vi "test Future Already Completed if Resolved after Timeout.vi"(8 "error in (no error)":errorcluster, 11 "TestCase in":refnum<class "Result Tests.lvclass">) -> (0 "error out":errorcluster, 3 "TestCase out":refnum<class "Result Tests.lvclass">)   [LabVIEW 2017, in "Result Tests.lvclass"]
uses:
  Result Tests.lvclass
  <vilib>/addons/_JKI Toolkits/VI Tester/TestCase.llb/TestCase.lvclass
  Futures/Result/Result.lvclass
  C:/Program Files (x86)/National Instruments/LabVIEW 2017/vi.lib/addons/_JKI Toolkits/VI Tester/TestCase.llb/TestCase.lvclass
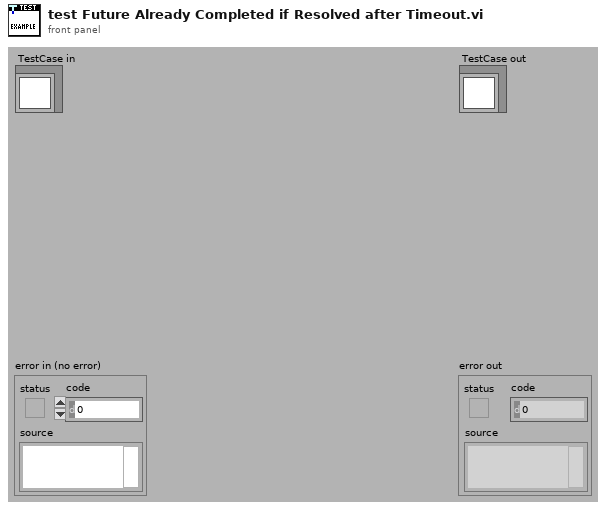
[diagram p1: front panel]
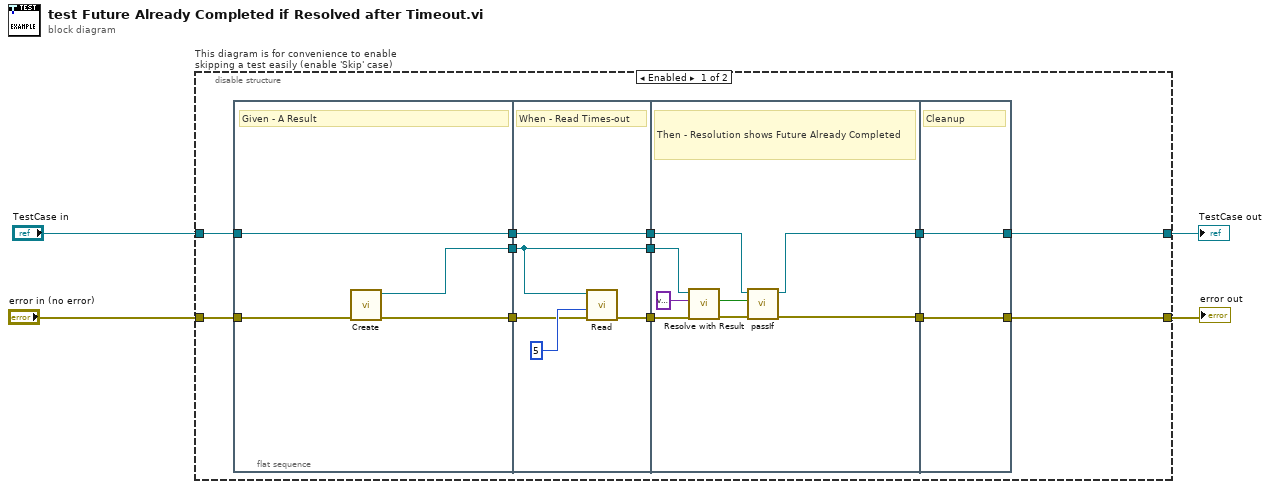
[diagram p0: block diagram]
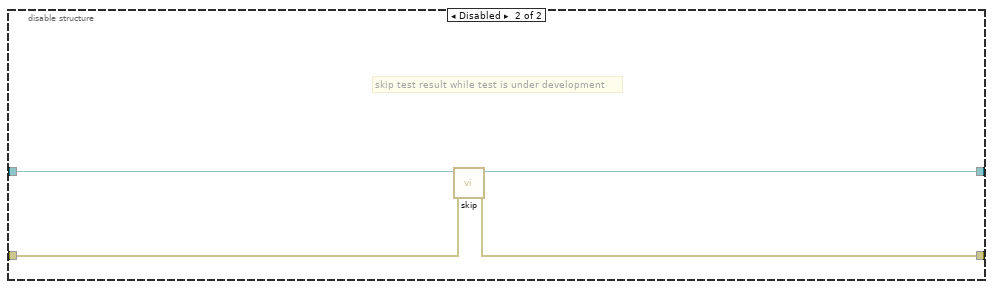
[diagram p2: hidden frame]
diagram:
  n1 = disable-structure "This diagram is for convenience to enable skipping a test easily (enable 'Skip' case)" shown="Enabled" {
    disable-tunnel: "TestCase in" -> [w11 w39]
    disable-tunnel: [w9 w37] -> w1
    disable-tunnel: [w8 w38] -> w3
    disable-tunnel: "error in (no error)" -> [w10 w36]
    frame Enabled {
      n2 = flat-sequence {
        tunnel: w10 -> [w19]
        tunnel: w11 -> [w20]
        tunnel: [w20] -> w16
        tunnel: [w18] -> w15
        tunnel: [w17] -> w7
        tunnel: [w25] -> w14
        tunnel: w16 -> [w25]
        tunnel: w15 -> [w23]
        tunnel: w7 -> [w21]
        tunnel: [w22] -> w6
        tunnel: [w21] -> w5
        tunnel: [w27] -> w13
        tunnel: [w28] -> w12
        tunnel: w14 -> [w29]
        tunnel: w6 -> [w32]
        tunnel: w5 -> [w33]
        tunnel: [w34] -> w8
        tunnel: [w35] -> w9
        tunnel: w13 -> [w35]
        tunnel: w12 -> [w34]
        frame #0 {
          # "Given - A Result"
          n3 = call "Create.vi"("error in (no error)"=w19) -> ("error out"=w18:errorcluster, "Result out"=w17:refnum<class "Result.lvclass">)  [unwired: 9 in]
        }
        frame #1 {
          # "When - Read Times-out"
          n4 = call "Read.vi"("error in (no error)"=w23, "timeout in ms (60 sec)"=5, "Result in"=w21) -> ("error out"=w22:errorcluster)  [unwired: 4 in, 4 out]
        }
        frame #2 {
          # "Then - Resolution shows Future Already Completed"
          n5 = call "Resolve with Result.vi"("error in (no error)"=w32, "Result"=variant, "Result in"=w33) -> ("error out"=w30:errorcluster, "Future Already Completed"=w31:bool)  [unwired: 6 in, 1 out]
          n6 = call-dynamic "passIf.vi"("error in (no error)"=w30, "pass"=w31, "TestCase in"=w29) -> ("error out"=w28:errorcluster, "TestCase out"=w27:refnum<class "Result Tests.lvclass">)  [unwired: 7 in]
        }
        frame #3 {
          # "Cleanup"
        }
      }
    }
    frame Disabled {
      # "skip test result while test is under development"
      n7 = call <vilib>:"skip.vi"("error in (no error)"=w36, "TestCase in"=w39) -> ("error out"=w38:errorcluster, "TestCase out"=w37:refnum<class "Result Tests.lvclass">)  [unwired: 8 in]
    }
  }
  "error out" <- w3
  "TestCase out" <- w1
